vi "Minibot Activate.vi"(11 "Fire Minibot":bool) -> ()   [LabVIEW 2012]
uses:
  <vilib>/Rock Robotics/WPI/Solenoid/WPI_SolenoidValue.ctl
  <vilib>/Rock Robotics/WPI/Solenoid/WPI_SolenoidSetEnum.vi
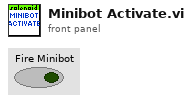
[diagram p1: front panel]
types:
  T1 = typedef "WPI_SolenoidValue.ctl" = enum16{"Off", "On", "Forward", "Reverse"}
  T2 = typedef "WPI_SolenoidDevRef.ctl" = cluster{"DevStatus":errorcluster, "Solenoid Module":T3, "Forward Solenoid Channel":T4, "Reverse Solenoid Channel":T4}
  T3 = typedef "FPGA_TypedefSolenoidModule.ctl" = enum16{"Solenoid Module 1", "Solenoid Module 2"}
  T4 = typedef "WPI_SolenoidChannel.ctl" = enum8{"Solenoid 1", "Solenoid 2", "Solenoid 3", "Solenoid 4", "Solenoid 5", "Solenoid 6", "Solenoid 7", "Solenoid 8", "Invalid"}
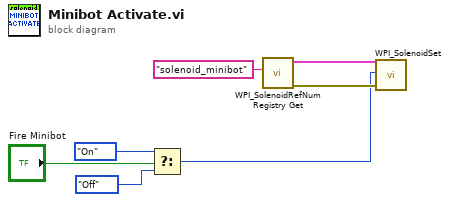
[diagram p0: block diagram]
diagram:
  n1 = Select(t=WPI_SolenoidValue."On" ("Value"), s="Fire Minibot", f=WPI_SolenoidValue."Off") -> (s? t:f=w2:T1)
  n2 = call <vilib>:"WPI_SolenoidRefNum Registry Get.vi"("refnum name"="solenoid_minibot") -> ("error out"=w6:errorcluster, "SolenoidDevRef"=w7:T2)  [unwired: 9 in]
  n3 = call-poly <vilib>:"WPI_SolenoidSet.vi"("error in (no error)"=w6, "Value"=w2, "SolenoidDevRef"=w7) -> ()  [unwired: 7 in, 2 out]
